vi "Example Callback - Count Callback.vi"(4 "Count":refnum<user-event>, 5 "Event Data":cluster{"sender":refnum<k24>, "count":i32}, 6 "Control Ref":refnum<k24>, 7 "Event Common Data":T1) -> ()   [LabVIEW 2010]
uses:
  C:/tf/play/labview/Tinkerforge.dll
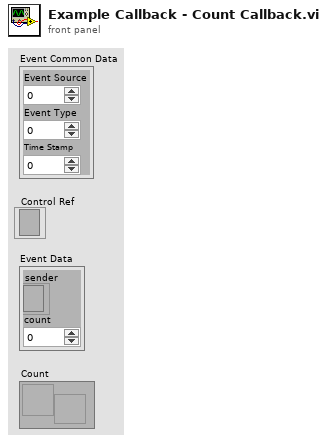
[diagram p1: front panel]
types:
  T1 = cluster{"Event Source":i32, "Event Type":u32, "Time Stamp":u32}
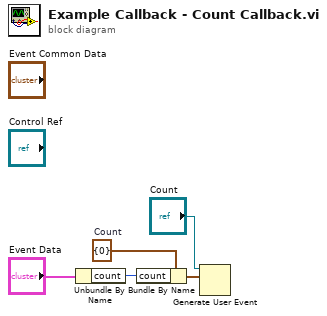
[diagram p0: block diagram]
diagram:
  w3 = cluster{"count":i32} {"count"=0}  # Count
  n1 = Unbundle By Name("Event Data") -> ("count"=w2:i32)
  n2 = Bundle By Name(cluster=w3, "count"=w2) -> (w4:cluster{"count":i32})
  n3 = Generate User Event(user event="Count", event data cluster=w4) -> ()  [unwired: 1 in, 2 out]
